vi "ExecuteItem.vi"(8 "error in (no error)":errorcluster, 10 "Tag":string, 11 "TreeControl in":refnum<vi>) -> (0 "error out":errorcluster)   [LabVIEW 2021, in "ScriptManager.lvlib"]
uses:
  ScriptManager.lvlib
  lib/SetGetControlValue/SetGetControlValue.lvlib
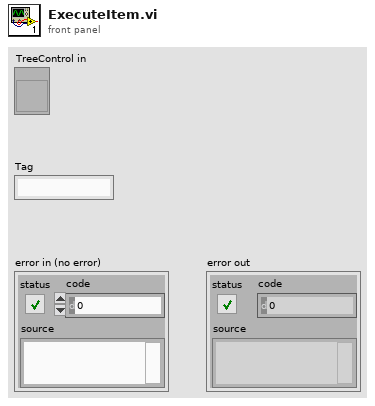
[diagram p1: front panel]
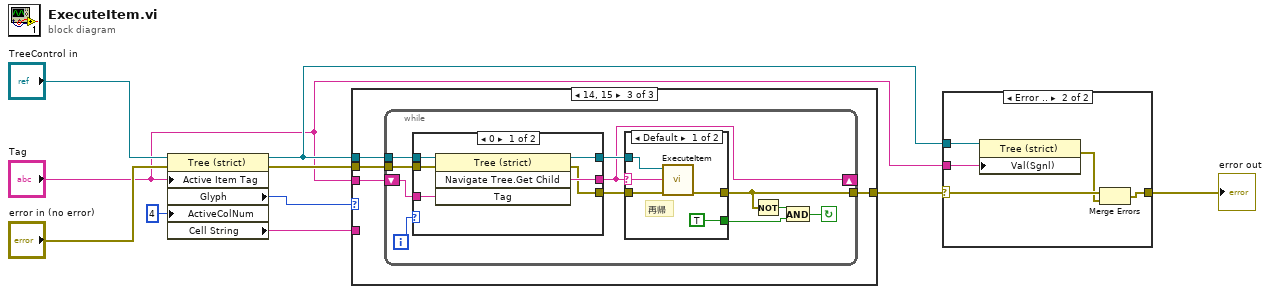
[diagram p0: block diagram]
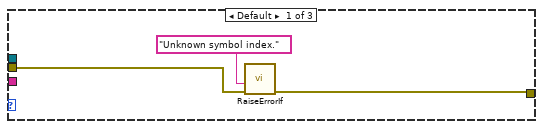
[diagram p3: hidden frame]
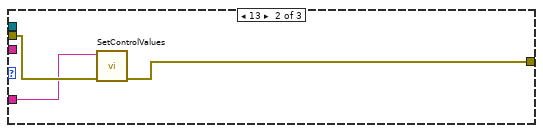
[diagram p4: hidden frame]
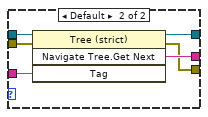
[diagram p6: hidden frame]
diagram:
  n1 = property class="Tree (strict)"(reference="TreeControl in", error in="error in (no error)", "Active Item Tag"="Tag", "ActiveColNum"=4 ("Active Cell:Active Column Number")) -> (reference out=w3:refnum<vi>, error out=w7:errorcluster, "Glyph"=w8:i32, "Cell String"=w1:string)
  n2 = case shown="14, 15" w8 {
    tunnel: w3 -> [_ _ w20]
    tunnel: w7 -> [w12 w16 w19]
    tunnel: "Tag" -> [_ _ w18]
    tunnel: [w13 w15 w17] -> w5
    tunnel: w1 -> [_ w14 _]
    frame Default {
      n3 = call "RaiseErrorIf.vi"("error in (no error)"=w12, "error message"="Unknown symbol index.") -> ("error out"=w13:errorcluster)  [unwired: 9 in]
    }
    frame 13 {
      n4 = call "SetControlValues.vi"("error in"=w16, "ControlValueList"=w14) -> ("error out"=w15:errorcluster)  [unwired: 9 in]
    }
    frame 14, 15 {
      n5 = while {
        tunnel: w20 -> [w31]
        tunnel: w19 -> [w30]
        tunnel: [w25] -> w17
        shift-right: [w21] -> _
        shift-left: w18 -> [w29]
        i -> [w28]
        stop <- w22 continue-if-true
        n6 = case shown="0" w28 {
          tunnel: w31 -> [w43 w49]
          tunnel: w30 -> [w42 w48]
          tunnel: w29 -> [w41 w47]
          tunnel: [w40 w46] -> w21
          tunnel: [w38 w45] -> w27
          tunnel: [w39 w44] -> w26
          frame 0 {
            n7 = invoke class="Tree (strict)" method="Navigate Tree.Get Child"(reference=w43, error in=w42, "Tag"=w41) -> (reference out=w38:refnum<vi>, error out=w39:errorcluster, "Navigate Tree:Get Child"=w40:string)  [unwired: 1 in, 1 out]
          }
          frame Default {
            n8 = invoke class="Tree (strict)" method="Navigate Tree.Get Next"(reference=w49, error in=w48, "Tag"=w47) -> (reference out=w45:refnum<vi>, error out=w44:errorcluster, "Navigate Tree:Get Next Item"=w46:string)  [unwired: 1 in, 1 out]
          }
        }
        n9 = case shown="Default" w21 {
          selector: w21 -> [w35 _]
          tunnel: w27 -> [w36 _]
          tunnel: w26 -> [w34 w37]
          tunnel: [w33 w37] -> w25
          tunnel: [TRUE _] -> w23
          frame Default {
            # "再帰"
            n10 = call "ExecuteItem.vi"("error in (no error)"=w34, "Tag"=w35, "TreeControl in"=w36) -> ("error out"=w33:errorcluster)  [unwired: 8 in]
          }
          frame "" {
          }
        }
        n11 = Not(x=w25) -> (.not. x?=w24:bool)
        n12 = And(x=w24, y=w23) -> (x .and. y?=w22:bool)
      }
    }
  }
  n13 = case shown="Error .." w5 {
    selector: w5 -> [w50 w52]
    tunnel: [w50 w53] -> w4
    tunnel: w3 -> [_ w55]
    tunnel: "Tag" -> [_ w54]
    frame No Error {
    }
    frame Error {
      n14 = property class="Tree (strict)"(reference=w55, "Val(Sgnl)"=w54) -> (error out=w51:errorcluster)  [unwired: 1 in, 1 out]
      n15 = Merge Errors(w52, w51) -> (w53:errorcluster)
    }
  }
  "error out" <- w4
